vi "详细故障分解.vi"(3 "名称":string[](array[string]), 5 "故障输入口":string[](array[string])) -> (0 "故障等级":dbl, 1 "输出数组":string[][](array[string]), 2 "故障显示":string[][](array[string]))   [LabVIEW 2013]
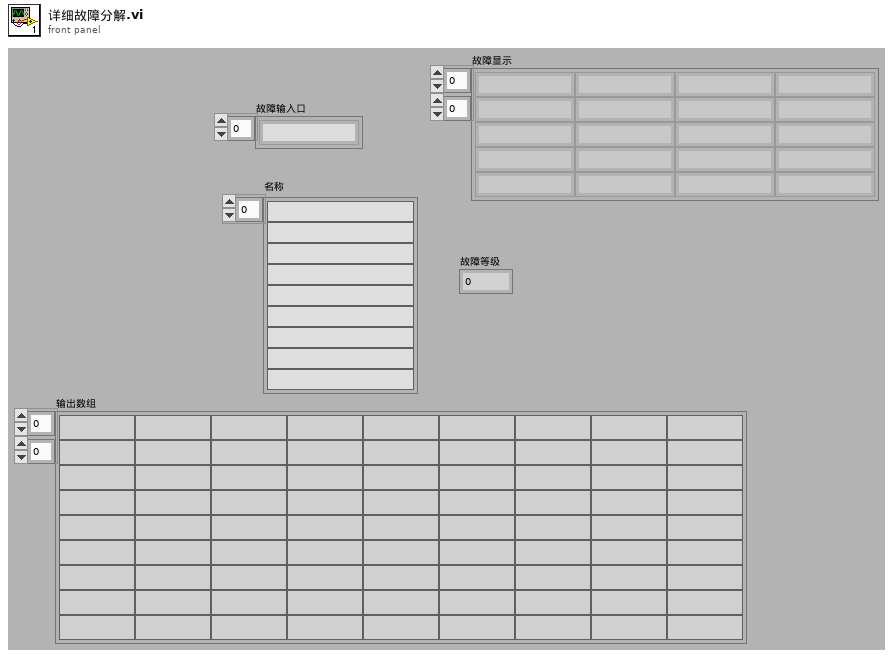
[diagram p1: front panel]
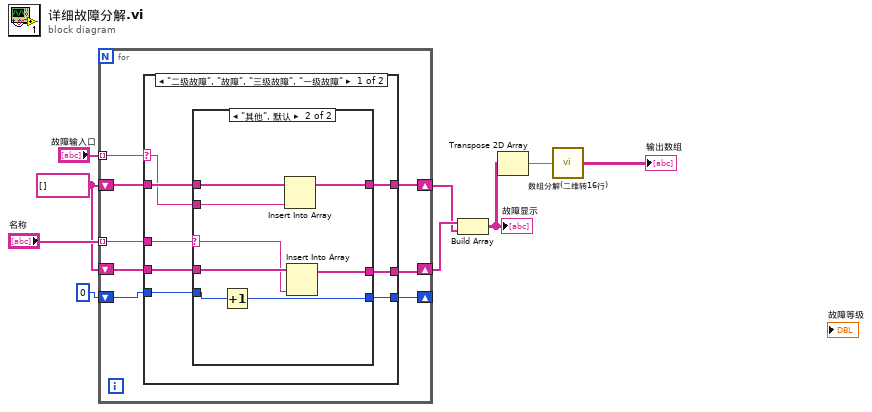
[diagram p0: block diagram]
diagram:
  w8 = string[] []
  n1 = for {
    tunnel: "故障输入口" -> [w17] mode=indexing
    tunnel: "名称" -> [w14] mode=indexing
    shift-right: [w16] -> w4
    shift-left: w8 -> [w15]
    shift-right: [w12] -> w5
    shift-left: w8 -> [w13]
    shift-right: [w10] -> _
    shift-left: 0 ("数值") -> [w11]
    n2 = case shown="\"二级故障\", \"故障\", \"三级故障\", \"一级故障\"" w17 {
      selector: w17 -> [w23 _]
      tunnel: [w25 w39] -> w16
      tunnel: w15 -> [w24 w39]
      tunnel: w14 -> [w22 _]
      tunnel: w13 -> [w21 w38]
      tunnel: [w20 w38] -> w12
      tunnel: w11 -> [w19 w37]
      tunnel: [w18 w37] -> w10
      frame "二级故障", "故障", "三级故障", "一级故障" {
        n3 = case shown="\"其他\", 默认" w22 {
          selector: w22 -> [_ w31]
          tunnel: [w28 w36] -> w25
          tunnel: w24 -> [w28 w35]
          tunnel: w23 -> [_ w34]
          tunnel: w21 -> [w27 w33]
          tunnel: [w27 w32] -> w20
          tunnel: [w26 w29] -> w18
          tunnel: w19 -> [w26 w30]
          frame "保留" {
          }
          frame "其他", Default {
            n4 = Increment(x=w30) -> (x+1=w29:i32)
            n5 = Insert Into Array(array=w35, new element=w34) -> (w36:string[])  [unwired: 1 in]
            n6 = Insert Into Array(array=w33, new element=w31) -> (w32:string[])  [unwired: 1 in]
          }
        }
      }
      frame "无故障", Default {
      }
    }
  }
  n7 = Build Array(w5, w4) -> (w6:string[][])
  "故障显示" <- w6
  n8 = Transpose 2D Array(2D array=w6) -> (transposed array=w2:string[][])
  n9 = call "数组分解(二维转16行).vi"("输入数组"=w2) -> ("输出数组"=→"输出数组":string[][])
